vi "Format Physical Channel.vi"(9 "Channel":i32, 10 "DAQmx Task prefix":string, 11 "Alias":string) -> (1 "Physical Channel":string)   [LabVIEW 2021, in "Load Frame.lvlib"]
doc: "Create a DAQmx Physical Channel expression using 'Alias', 'DAQmx Task prefix', and 'Channel'."
uses:
  Load Frame.lvlib
panel:
  in  "error in (no error)":errorcluster
  out "error out":errorcluster
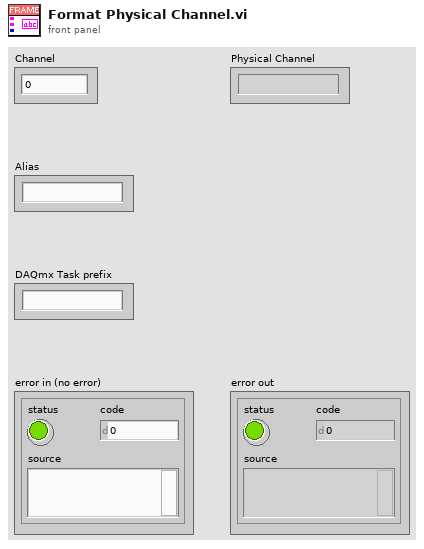
[diagram p1: front panel]
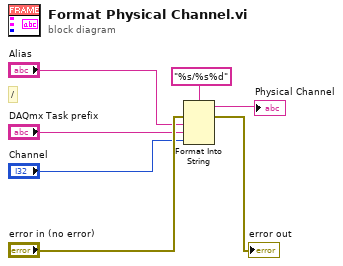
[diagram p0: block diagram]
diagram:
  # "/"
  n1 = Format Into String(format string="%s/%s%d", error in="error in (no error)", "Alias", "DAQmx Task prefix", "Channel") -> (resulting string=→"Physical Channel":string, error out=→"error out":errorcluster)  [unwired: 1 in]
